vi "AalborgDFCCommand.vi"(4 "Channel Name":string="Aalborg", 6 "Port Name":string="mfc1", 7 "Timeout/ms":u32=1500, 8 "Numeric Value":dbl format="%.6g", 9 "AalborgDFCCommand":T2="FullScaleRatingSLPM", 10 "Address":u8) -> (0 "String Reply":string="!11,100.0000\r\n", 1 "Error Description":string, 2 "Numeric Reply":dbl=100.0 format="%_6g", 3 "OK":bool)   [LabVIEW 2021]
uses:
  AalborgDFCCommand.ctl
  AalborgDFCCommandDescriptor.ctl
  AalborgDFCCommandPhases.ctl
panel:
  out "commandString":string
  out "Audit trail":string[](array[string])
  out "CommandDescriptorOutput":T1={"Command"="FullScaleRatingSLPM", "Mnemonic"="E", "Min"=nan, "Max"=nan, "ActionPath"=["PassCommand", "Communicate", "ParseNumber", "Done"]}
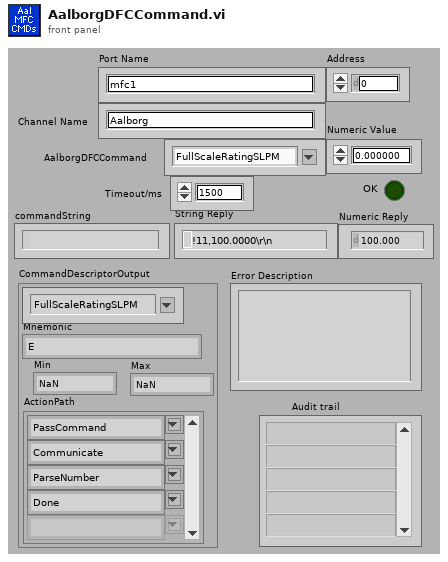
[diagram p1: front panel]
types:
  T1 = typedef "AalborgDFCCommandDescriptor.ctl" = cluster{"Command":T2, "Mnemonic":string, "Min":dbl, "Max":dbl, "ActionPath":T3[]}
  T2 = typedef "AalborgDFCCommand.ctl" = string
  T3 = typedef "AalborgDFCCommandPhases.ctl" = string
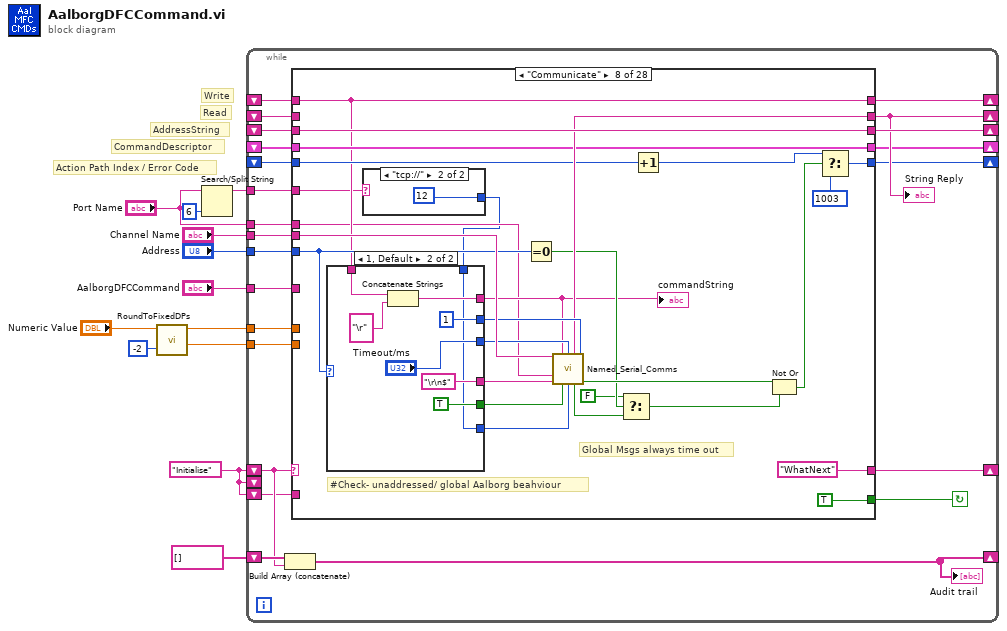
[diagram p0: block diagram]
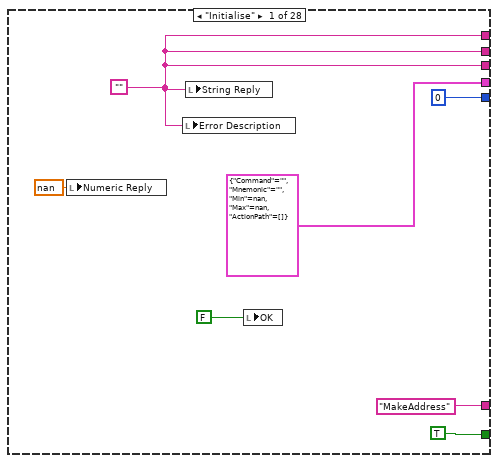
[diagram p2: hidden frame]
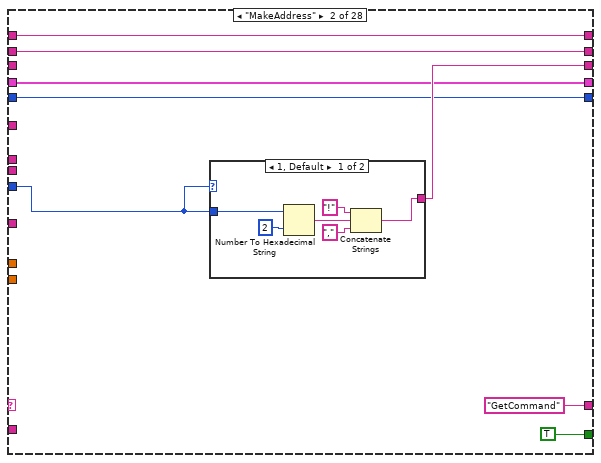
[diagram p3: hidden frame]
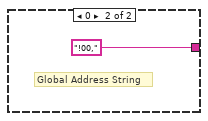
[diagram p4: hidden frame]
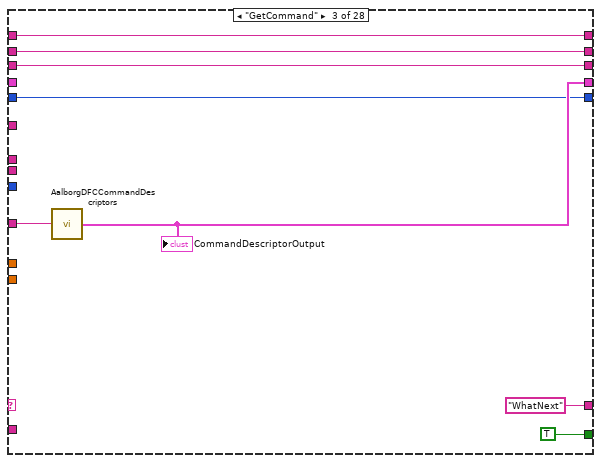
[diagram p5: hidden frame]
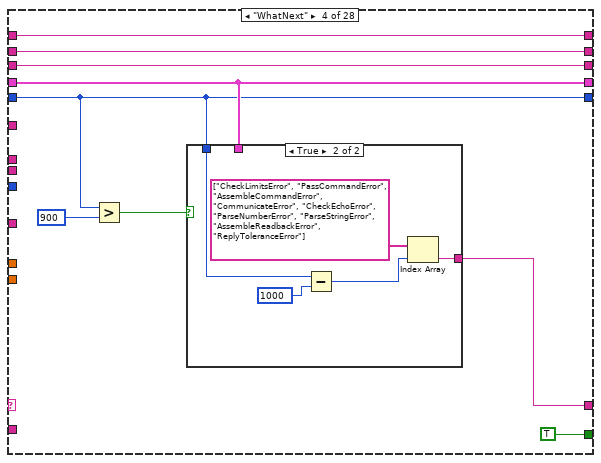
[diagram p6: hidden frame]
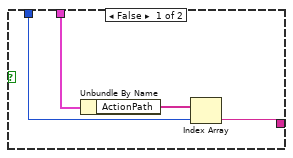
[diagram p7: hidden frame]
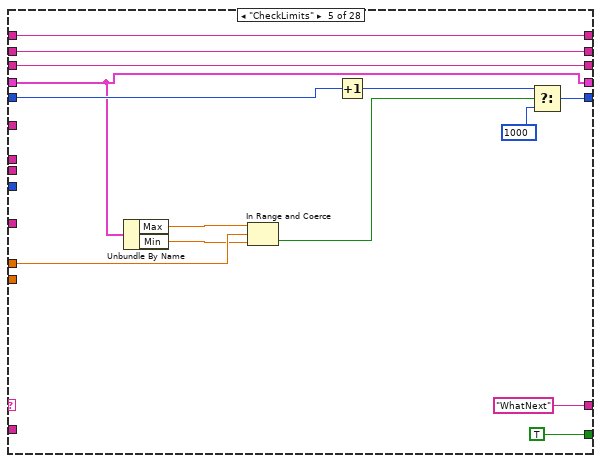
[diagram p8: hidden frame]
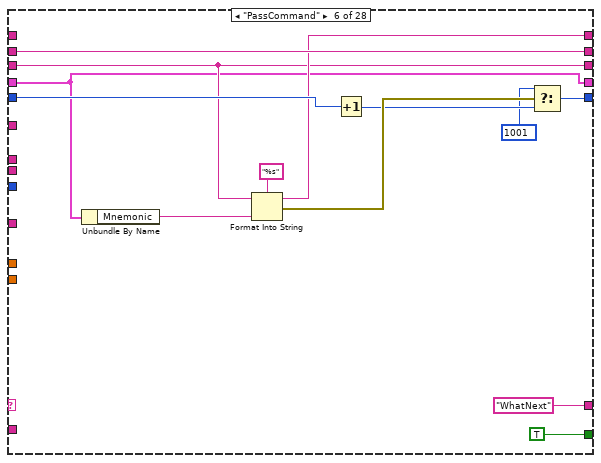
[diagram p9: hidden frame]
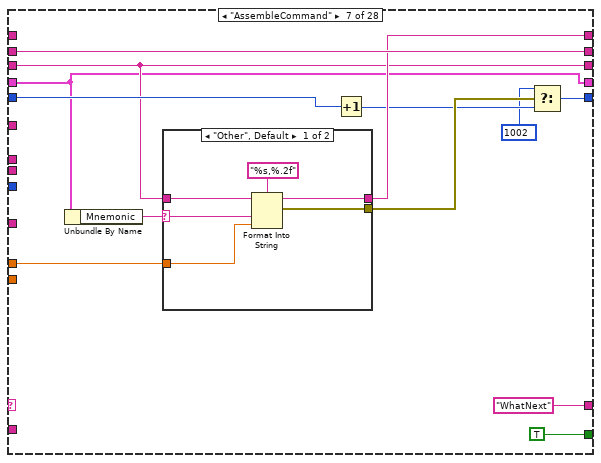
[diagram p10: hidden frame]
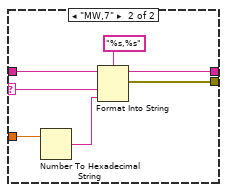
[diagram p11: hidden frame]
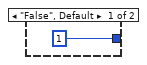
[diagram p12: hidden frame]
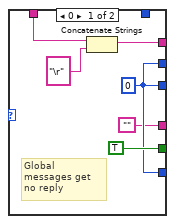
[diagram p13: hidden frame]
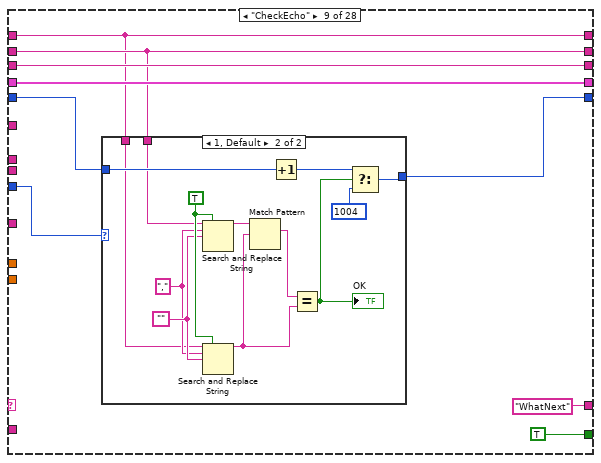
[diagram p14: hidden frame]
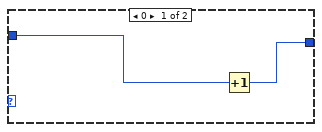
[diagram p15: hidden frame]
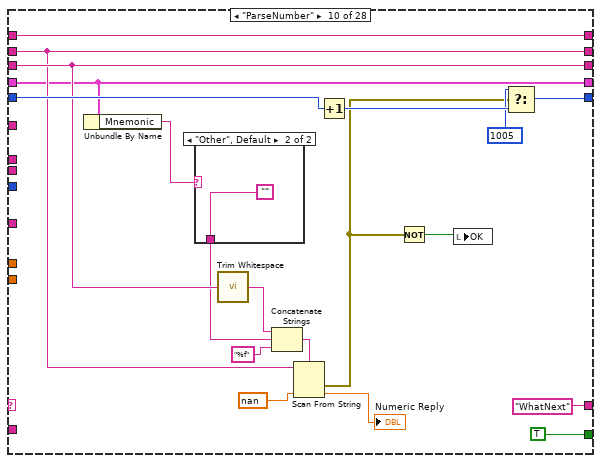
[diagram p16: hidden frame]
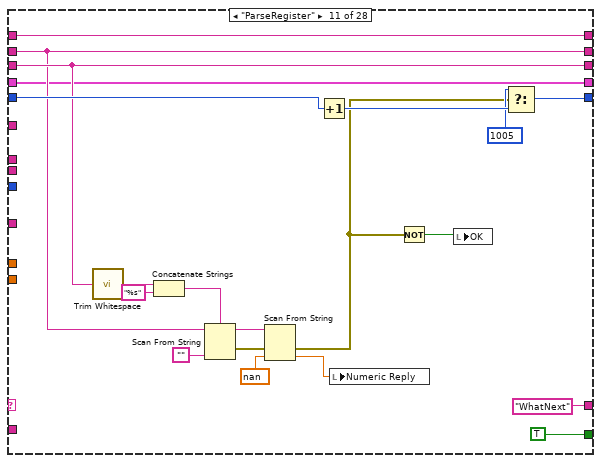
[diagram p18: hidden frame]
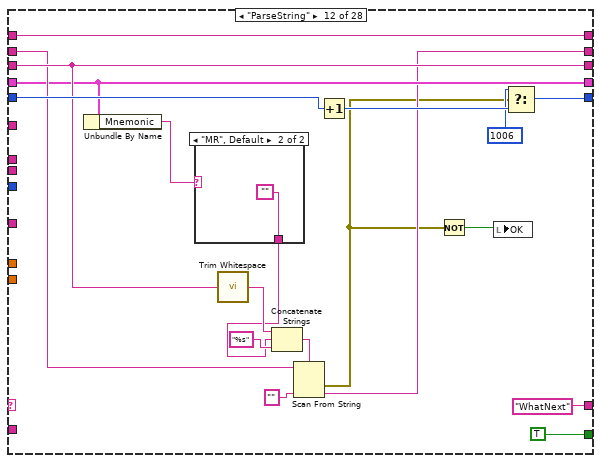
[diagram p19: hidden frame]
diagram:
  w8 = "Initialise"
  # "Action Path Index / Error Code"
  # "CommandDescriptor"
  # "AddressString"
  # "Read"
  # "Write"
  n1 = call "RoundToFixedDPs.vi"("Power of ten"=-2, "Number to round"="Numeric Value") -> ("Decimal place"=w4:dbl, "Rounded number"=w5:dbl)  [unwired: 8 in]
  n2 = Search/Split String(string="Port Name", offset (0)=6) -> (substring before match=w1:string)  [unwired: 1 in, 2 out]
  n3 = while {
    shift-right: [w23] -> _
    shift-left: w8 -> [w17]
    tunnel: "Address" -> [w35]
    tunnel: "AalborgDFCCommand" -> [w34]
    tunnel: w5 -> [w33]
    shift-right: [w32] -> _
    shift-left: _ -> [w31]
    tunnel: "Port Name" -> [w30]
    tunnel: "Channel Name" -> [w29]
    shift-right: [w22] -> _
    shift-left: _ -> [w28]
    shift-right: [w26] -> _
    shift-left: _ -> [w25]
    shift-right: [w15] -> _
    shift-left: string[] [] -> [w24]
    shift-right: [w21] -> _
    shift-left: _ -> [w20]
    shift-right: [w18] -> _
    shift-left: _ -> [w19]
    shift-left: w8 -> [_]
    shift-left: w8 -> [w16]
    tunnel: w4 -> [w14]
    tunnel: w1 -> [w13]
    stop <- w27 continue-if-true
    n4 = Build Array (concatenate)(w24, w17) -> (w15:T3[])
    "Audit trail" <- w15
    n5 = case shown="\"Communicate\"" w17 {
      selector: w17 -> [_ _ _ _ _ _ _ _ _ _ _ _ _ _ _ _ _ _ _ _ _ _ _ _ _ _ _ w478]
      tunnel: ["MakeAddress" "GetCommand" "WhatNext" w70 "WhatNext" "WhatNext" "WhatNext" "WhatNext" "WhatNext" "WhatNext" "WhatNext" "WhatNext" "WhatNext" "WhatNext" w314 "Error" "Initialise" "Error" "Error" "Error" "Error" "Error" "Error" "Error" "Error" "Error" "Error" w478] -> w23
      tunnel: w35 -> [_ w43 _ _ _ _ _ w142 w180 _ _ _ w269 _ _ _ _ w366 w377 w387 w398 w408 w421 w432 w443 w454 w463 _]
      tunnel: w34 -> [_ _ w62 _ _ _ _ _ _ _ _ _ _ _ _ _ _ _ _ _ _ _ _ _ _ _ _ _]
      tunnel: w33 -> [_ _ _ _ w95 _ w111 _ _ _ _ _ _ w287 _ _ _ w369 _ w390 _ _ _ _ _ _ _ _]
      tunnel: [w37 w48 w64 w73 w93 w105 w118 w141 w181 w214 w238 w254 w272 w293 w320 w336 w348 w374 w384 w395 w405 w417 w429 w440 w451 w460 w471 w476] -> w32
      tunnel: w31 -> [_ w48 w64 w73 w93 _ _ w141 w181 w214 w238 w254 _ w293 w320 w336 w358 _ _ _ _ w411 w423 _ _ _ _ _]
      tunnel: w30 -> [_ _ _ _ _ _ _ w139 _ _ _ _ _ _ _ _ w359 _ _ _ _ _ _ _ _ _ _ _]
      tunnel: w29 -> [_ _ _ _ _ _ _ w163 _ _ _ _ _ _ _ w331 w360 _ _ _ _ _ _ _ _ _ _ _]
      tunnel: [w37 w47 w63 w72 w97 w110 w123 w155 w182 w212 w236 w247 w277 w300 w318 w341 w349 w374 w384 w395 w405 w417 w420 w440 w451 w460 w471 w476] -> w22
      tunnel: w28 -> [_ w47 w63 w72 w97 w110 w123 _ w182 w212 w236 w252 w277 w300 w318 w341 w349 _ _ _ _ w410 w420 w434 w445 _ w465 _]
      tunnel: [TRUE TRUE ("Continue") TRUE ("Continue") TRUE ("Continue") TRUE TRUE TRUE TRUE TRUE TRUE TRUE TRUE TRUE TRUE w315 TRUE w350 TRUE ("Continue") TRUE ("Continue") TRUE ("Continue") TRUE ("Continue") TRUE ("Continue") TRUE ("Continue") TRUE ("Continue") TRUE ("Continue") TRUE ("Continue") TRUE ("Continue") FALSE] -> w27
      tunnel: [w37 w50 w61 w71 w96 w104 w117 w156 w187 w213 w237 w253 w270 w295 w319 w346 w348 w374 w384 w395 w405 w417 w429 w440 w451 w460 w471 w476] -> w26
      tunnel: w25 -> [_ _ w61 w71 w96 w104 w117 w156 w187 w213 w237 w253 w270 w295 w319 w346 _ _ _ _ _ _ _ _ _ _ _ _]
      tunnel: [T1 {"Command"="", "Mnemonic"="", "Min"=nan, "Max"=nan, "ActionPath"=[]} ("CommandDescriptorOutput") w45 w59 w69 w84 w101 w116 w154 w183 w211 w235 w251 w268 w294 w312 w342 w364 w372 w382 w393 w403 w415 w427 w438 w449 w458 w469 w475] -> w21
      tunnel: w20 -> [_ w45 _ w69 w84 w101 w116 w154 w183 w211 w235 w251 w268 w294 w311 w342 w364 w372 w382 w393 w403 w415 w427 w438 w449 w458 w469 w475]
      tunnel: w19 -> [_ w44 w58 w68 w88 w106 w119 w149 w184 w219 w241 w260 w273 w296 _ w343 w363 w373 w383 w394 w404 w416 w428 w439 w450 w459 w470 w474]
      tunnel: [0 w44 w58 w68 w89 w107 w120 w151 w185 w220 w242 w261 w274 w297 0 ("f") w344 w363 w373 w383 w394 w404 w416 w428 w439 w450 w459 w470 w474] -> w18
      tunnel: w16 -> [_ _ _ _ _ _ _ _ _ _ _ _ _ _ _ _ w356 _ _ _ _ _ _ _ _ _ _ _]
      tunnel: w14 -> [_ _ _ _ _ _ _ _ _ _ _ _ _ w286 _ _ _ _ _ _ _ _ _ _ _ _ _ _]
      tunnel: w13 -> [_ _ _ _ _ _ _ w138 _ _ _ _ _ _ _ _ _ _ _ _ _ _ _ _ _ _ _ _]
      frame "Initialise" {
        w37 = ""
        n6 = local write "Numeric Reply"(nan ("Numeric Reply")) -> ()
        n7 = local write "Error Description"(w37) -> ()
        n8 = local write "String Reply"(w37) -> ()
        n9 = local write "OK"(FALSE ("GoodEcho")) -> ()
      }
      frame "MakeAddress" {
        n10 = case shown="1, Default" w43 {
          tunnel: w43 -> [w51 _]
          tunnel: [w52 "!00,"] -> w50
          frame 1, Default {
            n11 = Number To Hexadecimal String(1:i16 2 ("width (-)"), 2:w51) -> (0:w55:string)
            n12 = Concatenate Strings("!" ("string"), w55, "," ("string")) -> (w52:string)
          }
          frame 0 {
            # "Global Address String"
          }
        }
      }
      frame "GetCommand" {
        n13 = call "AalborgDFCCommandDescriptors.vi"("AalborgDFCCommand"=w62) -> ("CommandDescriptorOutput"=w59:T1)  [unwired: 4 out]
        "CommandDescriptorOutput" <- w59
      }
      frame "WhatNext" {
        n14 = Greater?(x=w68, y=900) -> (0:w66:bool)
        n15 = case shown="True" w66 {
          tunnel: [w77 w79] -> w70
          tunnel: w69 -> [w76 _]
          tunnel: w68 -> [w75 w82]
          frame False {
            n16 = Unbundle By Name(w76) -> ("ActionPath"=w78:T3[])
            n17 = Index Array(array=w78, index=w75) -> (element=w77:T3)
          }
          frame True {
            n18 = Subtract(x=w82, y=1000) -> (x-y=w80:i32)
            n19 = Index Array(array=string[] ["CheckLimitsError", "PassCommandError", "AssembleCommandError", "CommunicateError", "CheckEchoError", "ParseNumberError", "ParseStringError", "AssembleReadbackError", "ReplyToleranceError"], index=w80) -> (element=w79:string)
          }
        }
      }
      frame "CheckLimits" {
        n20 = Unbundle By Name(w84) -> ("Max"=w92:dbl, "Min"=w91:dbl)
        n21 = In Range and Coerce(upper limit=w92, x=w95, lower limit=w91) -> (In Range?=w86:bool)  [unwired: 1 out]
        n22 = Increment(x=w88) -> (x+1=w87:i32)
        n23 = Select(t=w87, s=w86, f=1000) -> (s? t:f=w89:i32)
      }
      frame "PassCommand" {
        n24 = Unbundle By Name(w101) -> ("Mnemonic"=w103:string)
        n25 = Format Into String(format string="%s", initial string=w104, w103) -> (resulting string=w105:string, error out=w100:errorcluster)  [unwired: 1 in]
        n26 = Increment(x=w106) -> (x+1=w99:i32)
        n27 = Select(t=1001 ("f"), s=w100, f=w99) -> (s? t:f=w107:i32)
      }
      frame "AssembleCommand" {
        n28 = Unbundle By Name(w116) -> ("Mnemonic"=w112:string)
        n29 = case shown="\"Other\", Default" w112 {
          selector: w112 -> [w124 w130]
          tunnel: [w129 w136] -> w118
          tunnel: w117 -> [w128 w135]
          tunnel: [w126 w133] -> w115
          tunnel: w111 -> [w125 w132]
          frame "Other", Default {
            n30 = Format Into String(format string="%s,%.2f", initial string=w128, w124, w125) -> (resulting string=w129:string, error out=w126:errorcluster)  [unwired: 1 in]
          }
          frame "MW,7" {
            n31 = Number To Hexadecimal String(2:w132) -> (0:w131:string)  [unwired: 1 in]
            n32 = Format Into String(format string="%s,%s", initial string=w135, w130, w131) -> (resulting string=w136:string, error out=w133:errorcluster)  [unwired: 1 in]
          }
        }
        n33 = Increment(x=w119) -> (x+1=w114:i32)
        n34 = Select(t=1002 ("f"), s=w115, f=w114) -> (s? t:f=w120:i32)
      }
      frame "Communicate" {
        # "#Check- unaddressed/ global Aalborg beahviour"
        # "Global Msgs always time out"
        n35 = case shown="\"tcp://\"" w138 {
          tunnel: [1 ("Terminate Count") 12 ("Terminate Count")] -> w137
          frame "False", Default {
          }
          frame "tcp://" {
          }
        }
        n36 = case shown="1, Default" w142 {
          tunnel: ["" "\r\n$"] -> w162
          tunnel: [w170 w172] -> w161
          tunnel: [w170 "Timeout/ms"] -> w160
          tunnel: [TRUE ("Log Errors?") TRUE ("Log Errors?")] -> w159
          tunnel: [w170 1 ("!Error retries")] -> w158
          tunnel: w141 -> [w167 w175]
          tunnel: [w168 w174] -> w140
          tunnel: w137 -> [_ w172]
          frame 0 {
            w170 = 0 ("!Error retries")
            # "Global messages get no reply"
            n37 = Concatenate Strings(w167, "\r" ("string")) -> (w168:string)
          }
          frame 1, Default {
            n38 = Concatenate Strings(w175, "\r" ("string")) -> (w174:string)
          }
        }
        "commandString" <- w140
        n39 = Equal To 0?(x=w142) -> (x = 0?=w145:bool)
        n40 = call "Named_Serial_Comms.vi"("Channel Name"=w163, "Write"=w140, "Timeout/ms"=w160, "!Error retries"=w158, "Port Name"=w139, "Term Grep"=w162, "Log Errors?"=w159, "Terminate Count"=w161) -> ("Read"=w155:string, "Timed out"=w144:bool, "Serial Error"=w152:bool)  [unwired: 1 in, 4 out]
        n41 = Select(t=FALSE, s=w145, f=w144) -> (s? t:f=w146:bool)
        n42 = Increment(x=w149) -> (x+1=w148:i32)
        n43 = Not Or(1:w146, 2:w152) -> (0:w150:bool)
        n44 = Select(t=w148, s=w150, f=1003) -> (s? t:f=w151:i32)
      }
      frame "CheckEcho" {
        n45 = case shown="1, Default" w180 {
          tunnel: [w189 w202] -> w185
          tunnel: w184 -> [w190 w200]
          tunnel: w182 -> [_ w193]
          tunnel: w181 -> [_ w192]
          frame 0 {
            n46 = Increment(x=w190) -> (x+1=w189:i32)
          }
          frame 1, Default {
            w194 = "," ("search string")
            w199 = TRUE ("replace all? (F)")
            w198 = ""
            n47 = Search and Replace String(replace all?=w199, input string=w193, search string=w194, replace string=w198) -> (result string=w197:string)  [unwired: 4 in, 3 out]
            n48 = Search and Replace String(replace all?=w199, input string=w192, search string=w194, replace string=w198) -> (result string=w195:string)  [unwired: 4 in, 3 out]
            n49 = Match Pattern(string=w197, regular expression=w195) -> (match substring=w196:string)  [unwired: 1 in, 3 out]
            n50 = Increment(x=w200) -> (x+1=w201:i32)
            n51 = Equal?(x=w196, y=w195) -> (x = y?=w191:bool)
            "OK" <- w191
            n52 = Select(t=w201, s=w191, f=1004) -> (s? t:f=w202:i32)
          }
        }
      }
      frame "ParseNumber" {
        n53 = Unbundle By Name(w211) -> ("Mnemonic"=w210:string)
        n54 = case shown="\"Other\", Default" w210 {
          selector: w210 -> [w223 _]
          tunnel: [w223 ""] -> w209
          frame "S" {
          }
          frame "Other", Default {
          }
        }
        n55 = call <vilib>:"Trim Whitespace.vi"("string"=w213) -> ("trimmed string"=w215:string)  [unwired: 1 in]
        n56 = Concatenate Strings(w215, w209, "%f" ("format string")) -> (w206:string)
        n57 = Scan From String(format string=w206, input string=w212, default 1=nan ("default value 1")) -> (error out=w208:errorcluster, output 1=→"Numeric Reply":dbl)  [unwired: 2 in, 2 out]
        n58 = Increment(x=w219) -> (x+1=w218:i32)
        n59 = Not(x=w208) -> (.not. x?=w207:bool)
        n60 = local write "OK"(w207) -> ()
        n61 = Select(t=1005, s=w208, f=w218) -> (s? t:f=w220:i32)
      }
      frame "ParseRegister" {
        n62 = call <vilib>:"Trim Whitespace.vi"("string"=w237) -> ("trimmed string"=w233:string)  [unwired: 1 in]
        n63 = Concatenate Strings(w233, "%s" ("string")) -> (w232:string)
        n64 = Scan From String(format string=w232, input string=w236, default 1="") -> (remaining string=w225:string, error out=w230:errorcluster)  [unwired: 2 in, 2 out]
        n65 = Scan From String(input string=w225, error in=w230, default 1=nan ("default value 1")) -> (error out=w229:errorcluster, output 1=w227:dbl)  [unwired: 2 in, 2 out]
        n66 = Increment(x=w241) -> (x+1=w240:i32)
        n67 = local write "Numeric Reply"(w227) -> ()
        n68 = Not(x=w229) -> (.not. x?=w234:bool)
        n69 = local write "OK"(w234) -> ()
        n70 = Select(t=1005, s=w229, f=w240) -> (s? t:f=w242:i32)
      }
      frame "ParseString" {
        n71 = Unbundle By Name(w251) -> ("Mnemonic"=w250:string)
        n72 = case shown="\"MR\", Default" w250 {
          selector: w250 -> [w264 _]
          tunnel: [w264 ""] -> w249
          frame "MW" {
          }
          frame "MR", Default {
          }
        }
        n73 = call <vilib>:"Trim Whitespace.vi"("string"=w253) -> ("trimmed string"=w255:string)  [unwired: 1 in]
        n74 = Concatenate Strings(w255, w249, "%s" ("format string")) -> (w257:string)
        n75 = Scan From String(format string=w257, input string=w252, default 1="") -> (error out=w245:errorcluster, output 1=w247:string)  [unwired: 2 in, 2 out]
        n76 = Increment(x=w260) -> (x+1=w259:i32)
        n77 = Not(x=w245) -> (.not. x?=w246:bool)
        n78 = local write "OK"(w246) -> ()
        n79 = Select(t=1006, s=w245, f=w259) -> (s? t:f=w261:i32)
      }
      frame "AssembleReadback" {
        n80 = case shown="1, Default" w269 {
          tunnel: w268 -> [_ w285]
          tunnel: ["" w284] -> w272
          tunnel: [errorcluster {"status"=TRUE, "code"=0, "source"=""} ("error IO") w283] -> w271
          tunnel: w270 -> [_ w282]
          frame 0 {
            # "Can't READ globally..."
          }
          frame 1, Default {
            # "#ToDo- Aalborg read value"
            n81 = Unbundle By Name(w285) -> ("Mnemonic"=w281:string)
            n82 = Format Into String(format string="PR %s\n", initial string=w282, w281) -> (resulting string=w284:string, error out=w283:errorcluster)  [unwired: 1 in]
          }
        }
        n83 = Increment(x=w273) -> (x+1=w266:i32)
        n84 = Select(t=1007 ("f"), s=w271, f=w266) -> (s? t:f=w274:i32)
      }
      frame "CompareReply" {
        # "-to avoid pesky floating point tiny differences!"
        n85 = local read "Numeric Reply"() -> (w292:dbl)
        n86 = Equal To 0?(x=w287) -> (x = 0?=w288:bool)
        n87 = case shown="False" w288 {
          tunnel: w292 -> [w308 w310]
          tunnel: w287 -> [w306 _]
          tunnel: [w304 w309] -> w289
          tunnel: w286 -> [w302 _]
          frame False {
            n88 = Subtract(x=w308, y=w306) -> (x-y=w307:dbl)
            n89 = Absolute Value(x=w307) -> (abs(x)=w305:dbl)
            n90 = Multiply(x=w302, y=1.01) -> (x*y=w303:dbl)
            n91 = Less Or Equal?(x=w305, y=w303) -> (x <= y?=w304:bool)
          }
          frame True {
            n92 = Equal To 0?(x=w310) -> (x = 0?=w309:bool)
          }
        }
        n93 = Increment(x=w296) -> (x+1=w290:i32)
        n94 = local write "OK"(w289) -> ()
        n95 = Select(t=w290, s=w289, f=1008) -> (s? t:f=w297:i32)
      }
      frame "Done" {
        # "#Check- What is the error prompt from Aalborgs?"
        n96 = Match Pattern(string=w318, regular expression="?") -> (offset past match=w313:i32)  [unwired: 4 out]
        n97 = case shown="0, Default" w313 {
          tunnel: [TRUE ("Continue") FALSE ("Continue")] -> w315
          tunnel: ["WhatNext" "Initialise"] -> w314
          tunnel: [w324 w325] -> w312
          tunnel: w311 -> [_ w325]
          frame 0, Default {
            # "#Check- What should we do \nif there's an error?"
            n98 = call "AalborgDFCCommandDescriptors.vi"("AalborgDFCCommand"=T2 "ValveStatus") -> ("CommandDescriptorOutput"=w324:T1)  [unwired: 4 out]
          }
          frame -1 {
          }
        }
      }
      frame "ParseError" {
        n99 = call <vilib>:"Trim Whitespace.vi"("string"=w336) -> ("trimmed string"=w334:string)  [unwired: 1 in]
        n100 = Concatenate Strings(w334, "%s" ("format string")) -> (w337:string)
        n101 = Scan From String(format string=w337, input string=w341, default 1="") -> (error out=w340:errorcluster, output 1=w332:string)  [unwired: 2 in, 2 out]
        n102 = call "AalborgDFCErrorCodes.vi"("Error Code"=w332) -> ("Error Description"=w330:string)  [unwired: 4 out]
        n103 = Increment(x=w343) -> (x+1=w339:i32)
        n104 = Format Into String(format string="The %s has %s", w331, w330) -> (resulting string=→"Error Description":string)  [unwired: 2 in, 1 out]
        n105 = Select(t=1007, s=w340, f=w339) -> (s? t:f=w344:i32)
      }
      frame "Error" {
        w353 = "Error in AalborgDFCCommand.vi: " ("string")
        w348 = ""
        w350 = FALSE ("Continue")
        n106 = local read "Error Description"() -> (w352:string)
        n107 = call "Serial_log_build.vi"("Read"=w349, "Write String"=w358, "Port Name"=w359) -> ("Output Array"=w361:string[])
        n108 = Empty String/Path?(string/path=w352) -> (empty?=w357:bool)
        n109 = Concatenate Strings(w353, w356) -> (w355:string)
        n110 = Concatenate Strings(w353, w352) -> (w354:string)
        n111 = Select(t=w355, s=w357, f=w354) -> (s? t:f=w351:string)
        n112 = call "Write_serial_log.vi"("Log Type"="AalborgDFC_Error_Log", "Log Array"=w361, "Header message"=w351, "Channel Name"=w360) -> ()  [unwired: 1 out]
        n113 = local write "OK"(w350) -> ()
      }
      frame "CheckLimitsError" {
        w374 = ""
        n114 = Unbundle By Name(w372) -> ("Mnemonic"=w370:string)
        n115 = Format Into String(format string="%s=%d) to MFC %x", initial string="Attempt to Write an out-of-range value (" ("message"), w370, w369, w366) -> (resulting string=w367:string)  [unwired: 1 in, 1 out]
        n116 = local write "Error Description"(w367) -> ()
      }
      frame "PassCommandError" {
        w384 = ""
        n117 = Unbundle By Name(w382) -> ("Mnemonic"=w380:string)
        n118 = Format Into String(format string="%s) to MFC %x", initial string="Attempt to PassCommand (" ("message"), w380, w377) -> (resulting string=w378:string)  [unwired: 1 in, 1 out]
        n119 = local write "Error Description"(w378) -> ()
      }
      frame "AssembleCommandError" {
        w395 = ""
        n120 = Unbundle By Name(w393) -> ("Mnemonic"=w391:string)
        n121 = Format Into String(format string="%s,%.1f) to MFC %x", initial string="Attempt to AssembleCommand (" ("message"), w391, w390, w387) -> (resulting string=w388:string)  [unwired: 1 in, 1 out]
        n122 = local write "Error Description"(w388) -> ()
      }
      frame "CommunicateError" {
        w405 = ""
        n123 = Unbundle By Name(w403) -> ("Command"=w401:T2)
        n124 = Format Into String(format string="%s) to MFC %x", initial string="Serial CommsError (" ("message"), w401, w398) -> (resulting string=w399:string)  [unwired: 1 in, 1 out]
        n125 = local write "Error Description"(w399) -> ()
      }
      frame "CheckEchoError" {
        w417 = ""
        n126 = Unbundle By Name(w415) -> ("Command"=w413:T2)
        n127 = Format Into String(format string="Command = %s; Write = %s; Read=%s) to MFC %x", initial string="Echo Error (" ("message"), w413, w411, w410, w408) -> (resulting string=w409:string)  [unwired: 1 in, 1 out]
        n128 = local write "Error Description"(w409) -> ()
      }
      frame "ReplyToleranceError" {
        w429 = ""
        n129 = Unbundle By Name(w427) -> ("Command"=w425:T2)
        n130 = Format Into String(format string="Command = %s; Write = %s; Read=%s) to MFC %x", initial string="Reply out of tolerance (" ("message"), w425, w423, w420, w421) -> (resulting string=w422:string)  [unwired: 1 in, 1 out]
        n131 = local write "Error Description"(w422) -> ()
      }
      frame "ParseNumberError" {
        w440 = ""
        n132 = Unbundle By Name(w438) -> ("Mnemonic"=w436:string)
        n133 = Format Into String(format string="%s=%s) from MFC %x", initial string="Attempt to ParseNumber (" ("message"), w436, w434, w432) -> (resulting string=w433:string)  [unwired: 1 in, 1 out]
        n134 = local write "Error Description"(w433) -> ()
      }
      frame "ParseStringError" {
        w451 = ""
        n135 = Unbundle By Name(w449) -> ("Mnemonic"=w447:string)
        n136 = Format Into String(format string="%s=%s) from MFC %x", initial string="Attempt to ParseString (" ("message"), w447, w445, w443) -> (resulting string=w444:string)  [unwired: 1 in, 1 out]
        n137 = local write "Error Description"(w444) -> ()
      }
      frame "AssembleReadbackError" {
        w460 = ""
        n138 = Format Into String(format string="to MFC %x", initial string="Attempt to AssembleReadback " ("message"), w454) -> (resulting string=w455:string)  [unwired: 1 in, 1 out]
        n139 = local write "Error Description"(w455) -> ()
      }
      frame "ParseErrorError" {
        w471 = ""
        n140 = Unbundle By Name(w469) -> ("Command"=w467:T2)
        n141 = Format Into String(format string="Command = %s; Read = %s) for MFC %x", initial string="Attempt to ParseError (" ("message"), w467, w465, w463) -> (resulting string=w464:string)  [unwired: 1 in, 1 out]
        n142 = local write "Error Description"(w464) -> ()
      }
      frame "NoMatch", Default {
        w476 = ""
        n143 = One Button Dialog(message="Case not found in AalborgDFCDriveCommand.vi", button name ("OK")="Shit!...") -> ()  [unwired: 1 out]
      }
    }
    "String Reply" <- w22
  }
